vi "_Sytem Status Manager.vi"(5 "Error IN":errorcluster, 8 "Action":T2) -> (14 "Status":T1, 19 "Error OUT":errorcluster)   [LabVIEW 2011]
uses:
  System Status Enum.ctl
  System Status Boolean.ctl
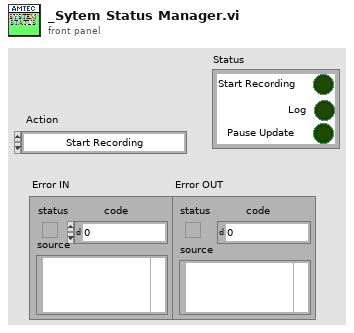
[diagram p1: front panel]
types:
  T1 = typedef "System Status Boolean.ctl" = cluster{"Start Recording":bool, "Log":bool, "Pause Update":bool}
  T2 = typedef "System Status Enum.ctl" = enum16{"Start Recording", "Stop Recording", "Log", "Stop Log", "Pause Update", "Resume Update", "Status", "Init"}
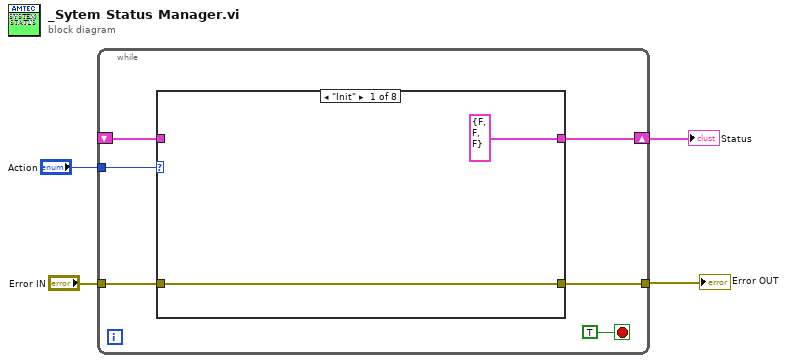
[diagram p0: block diagram]
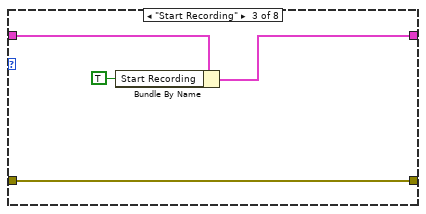
[diagram p3: hidden frame]
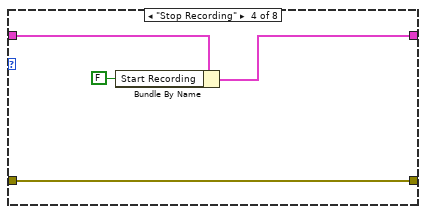
[diagram p4: hidden frame]
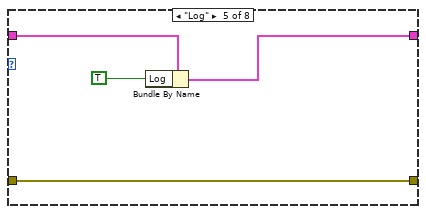
[diagram p5: hidden frame]
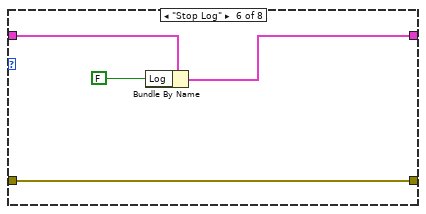
[diagram p6: hidden frame]
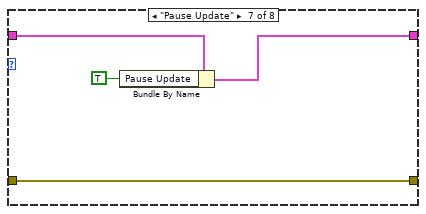
[diagram p7: hidden frame]
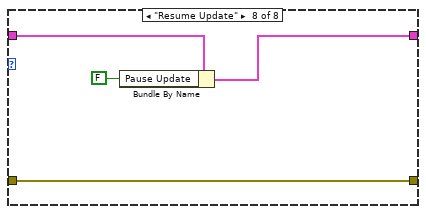
[diagram p8: hidden frame]
diagram:
  n1 = while {
    tunnel: "Action" -> [w9]
    tunnel: "Error IN" -> [w8]
    tunnel: [w7] -> w3
    shift-right: [w6] -> w1
    shift-left: _ -> [w5]
    stop <- TRUE stop-if-true
    n2 = case shown="\"Init\"" w9 {
      tunnel: w8 -> [w12 w14 w18 w22 w26 w30 w34 w38]
      tunnel: [w12 w14 w18 w22 w26 w30 w34 w38] -> w7
      tunnel: [T1 {"Start Recording"=FALSE, "Log"=FALSE, "Pause Update"=FALSE} ("Status") w13 w16 w20 w24 w28 w32 w36] -> w6
      tunnel: w5 -> [_ w13 w17 w21 w25 w29 w33 w37]
      frame "Init" {
      }
      frame "Status", Default {
      }
      frame "Start Recording" {
        n3 = Bundle By Name(cluster=w17, "Start Recording"=TRUE) -> (w16:T1)
      }
      frame "Stop Recording" {
        n4 = Bundle By Name(cluster=w21, "Start Recording"=FALSE) -> (w20:T1)
      }
      frame "Log" {
        n5 = Bundle By Name(cluster=w25, "Log"=TRUE ("Start Recording")) -> (w24:T1)
      }
      frame "Stop Log" {
        n6 = Bundle By Name(cluster=w29, "Log"=FALSE ("Start Recording")) -> (w28:T1)
      }
      frame "Pause Update" {
        n7 = Bundle By Name(cluster=w33, "Pause Update"=TRUE ("Start Recording")) -> (w32:T1)
      }
      frame "Resume Update" {
        n8 = Bundle By Name(cluster=w37, "Pause Update"=FALSE ("Start Recording")) -> (w36:T1)
      }
    }
  }
  "Error OUT" <- w3
  "Status" <- w1
